vi "set all flow rates.vi"(7 "background air flow rate":dbl, 8 "error in":errorcluster, 9 "dilution air flow rate":dbl, 10 "odor 1 flow rate":dbl, 11 "LabJack Tasks":T2) -> (0 "error out":errorcluster, 3 "flow rates":T3 {"pid reading" format="%0.2f"})   [LabVIEW 2021]
uses:
  temporal odor control/LabJack Interface/LabJack AOAI Channel.ctl
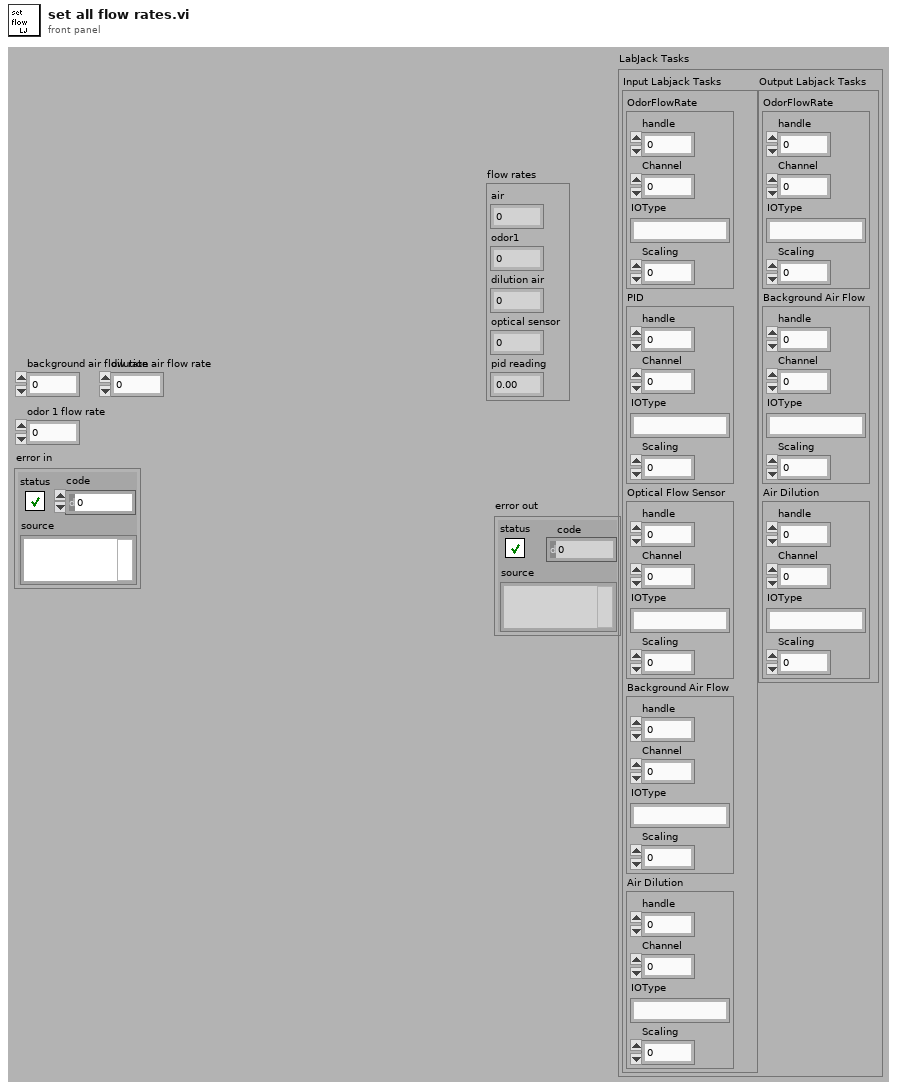
[diagram p1: front panel]
types:
  T1 = typedef "LabJack AOAI Channel.ctl" = cluster{"handle":i32, "Channel":i32, "IOType":string, "Scaling":dbl}
  T2 = cluster{"Input Labjack Tasks":cluster{"OdorFlowRate":T1, "PID":T1, "Optical Flow Sensor":T1, "Background Air Flow":T1, "Air Dilution":T1}, "Output Labjack Tasks":cluster{"OdorFlowRate":T1, "Background Air Flow":T1, "Air Dilution":T1}}
  T3 = cluster{"air":dbl, "odor1":dbl, "dilution air":dbl, "optical sensor":dbl, "pid reading":dbl}
  T4 = cluster{"OdorFlowRate":T1, "Background Air Flow":T1, "Air Dilution":T1}
  T5 = cluster{"OdorFlowRate":T1, "PID":T1, "Optical Flow Sensor":T1, "Background Air Flow":T1, "Air Dilution":T1}
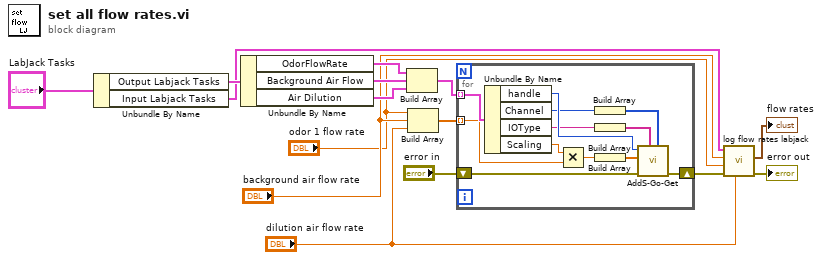
[diagram p0: block diagram]
diagram:
  n1 = Unbundle By Name("LabJack Tasks") -> ("Output Labjack Tasks"=w12:T4, "Input Labjack Tasks"=w5:T5)
  n2 = Unbundle By Name(w12) -> ("OdorFlowRate"=w11:T1, "Background Air Flow"=w10:T1, "Air Dilution"=w9:T1)
  n3 = Build Array(w11, w10, w9) -> (w8:T1[])
  n4 = Build Array("odor 1 flow rate", "background air flow rate", "dilution air flow rate") -> (w7:dbl[])
  n5 = for {
    tunnel: w8 -> [w27] mode=indexing
    tunnel: w7 -> [w25] mode=indexing
    shift-right: [w20] -> w1
    shift-left: "error in" -> [w21]
    n6 = Unbundle By Name(w27) -> ("handle"=w24:i32, "Channel"=w19:i32, "IOType"=w16:string, "Scaling"=w26:dbl)
    n7 = Multiply(x=w26, y=w25) -> (x*y=w23:dbl)
    n8 = Build Array(w19) -> (w18:i32[])
    n9 = Build Array(w16) -> (w17:string[])
    n10 = Build Array(w23) -> (w22:dbl[])
    n11 = call "AddS-Go-Get.vi"("Channels"=w18, "IOTypes"=w17, "error in"=w21, "Values Write"=w22, "Handle In"=w24) -> ("error out"=w20:errorcluster)  [unwired: 4 in, 2 out]
  }
  n12 = call "log flow rates labjack.vi"("Air Dilution Setpoint"="dilution air flow rate", "error in"=w1, "odor 1 setpoint"="odor 1 flow rate", "background air set point"="background air flow rate", "Input Labjack Tasks"=w5) -> ("error out"=→"error out":errorcluster, "flow rates"=→"flow rates":T3)  [unwired: 5 in]
